vi "SA_SWEEP_TIME.vi"(0 "Session In":refnum<visa-resource-name>="TCPIP0::K-N90X0A-00005.local::hislip0::INSTR", 1 "RO(F)":bool, 2 "Skip(F)":bool, 11 "error in":errorcluster {"code" format="%.0x"}, 12 "SetTime(ms)":u16=1, 13 "Timeout":u32=3000) -> (4 "Session Out":refnum<visa-resource-name>, 10 "GetTime(ms)":dbl, 15 "error out":errorcluster {"code" format="%.0x"})   [LabVIEW 2018]
doc: "Launches the Instrument I/O Assistant, which you can use to communicate with message-based instruments and graphically parse the response. For example you can communicate with an instrument that uses a serial, Ethernet, or GPIB interface."
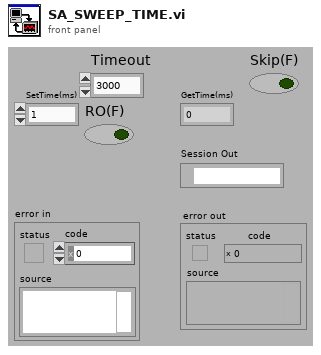
[diagram p1: front panel]
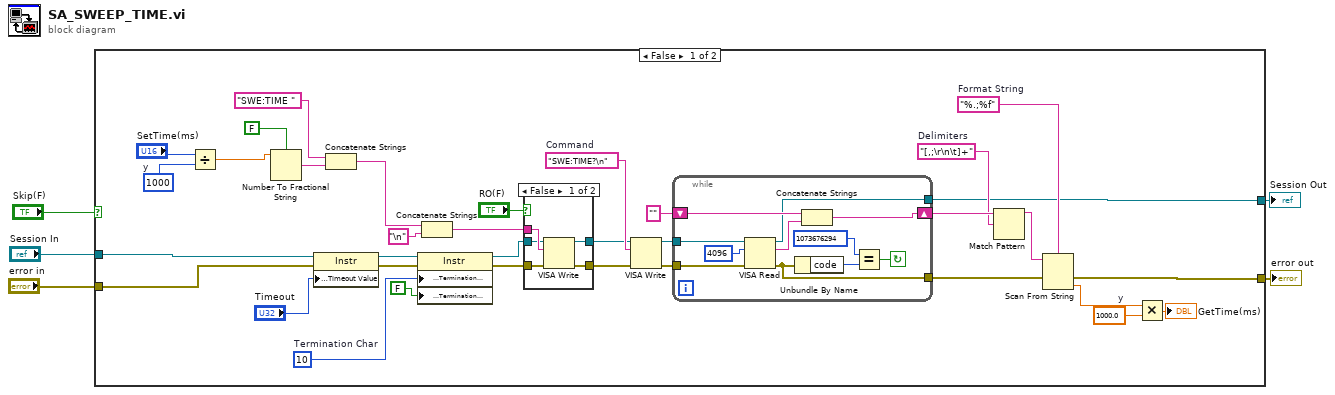
[diagram p0: block diagram]
diagram:
  n1 = case shown="False" "Skip(F)" {
    tunnel: "error in" -> [w40 w59]
    tunnel: "Session In" -> [w36 w60]
    tunnel: [w16 w59] -> w3
    tunnel: [w11 w60] -> w2
    frame False {
      w6 = 1000.0  # y
      w9 = u16 1000  # y
      w14 = "[,;\r\n\t]+"  # Delimiters
      w17 = "%.;%f"  # Format String
      w20 = "SWE:TIME?\n"  # Command
      w33 = u8 10  # Termination Char
      n2 = Divide(x="SetTime(ms)", y=w9) -> (x/y=w8:dbl)
      n3 = Number To Fractional String(use system decimal point (T)=FALSE, number=w8) -> (F-format string=w30:string)  [unwired: 2 in]
      n4 = property class="Instr"(reference=w36, error in=w40, "General Settings:Timeout Value"="Timeout") -> (reference out=w32:refnum<visa-resource-name>, error out=w35:errorcluster)
      n5 = Concatenate Strings("SWE:TIME " ("staticText"), w30) -> (w26:string)
      n6 = property class="Instr"(reference=w32, error in=w35, "Message Based Settings:Termination Character"=w33, "Message Based Settings:Termination Character Enable"=FALSE ("enable")) -> (reference out=w13:refnum<visa-resource-name>, error out=w34:errorcluster)
      n7 = Concatenate Strings(w26, "\n" ("StaticText")) -> (w27:string)
      n8 = case shown="False" "RO(F)" {
        tunnel: w34 -> [w45 w46]
        tunnel: [w44 w46] -> w28
        tunnel: w27 -> [w43 _]
        tunnel: w13 -> [w42 w47]
        tunnel: [w41 w47] -> w12
        frame False {
          n9 = VISA Write(VISA resource name=w42, write buffer=w43, error in (no error)=w45) -> (VISA resource name out=w41:refnum<visa-resource-name>, error out=w44:errorcluster)  [unwired: 1 out]
        }
        frame True {
        }
      }
      n10 = VISA Write(VISA resource name=w12, write buffer=w20, error in (no error)=w28) -> (VISA resource name out=w24:refnum<visa-resource-name>, error out=w23:errorcluster)  [unwired: 1 out]
      n11 = while {
        tunnel: w24 -> [w55]
        shift-right: [w49] -> w19
        shift-left: "" -> [w54]
        tunnel: w23 -> [w52]
        tunnel: [w51] -> w22
        tunnel: [w48] -> w11
        stop <- w50 continue-if-true
        n12 = VISA Read(VISA resource name=w55, byte count=u32 4096 ("byte count (0)"), error in (no error)=w52) -> (VISA resource name out=w48:refnum<visa-resource-name>, read buffer=w53:string, error out=w51:errorcluster)  [unwired: 1 out]
        n13 = Unbundle By Name(w51) -> ("code"=w57:i32)
        n14 = Concatenate Strings(w54, w53) -> (w49:string)
        n15 = Equal?(x=1073676294, y=w57) -> (x = y?=w50:bool)
      }
      n16 = Match Pattern(string=w19, regular expression=w14) -> (before substring=w18:string)  [unwired: 1 in, 3 out]
      n17 = Scan From String(format string=w17, input string=w18, error in=w22) -> (error out=w16:errorcluster, output 1=w15:dbl)  [unwired: 2 in, 2 out]
      n18 = Multiply(x=w15, y=w6) -> (x*y=→"GetTime(ms)":dbl)
    }
    frame True {
    }
  }
  "error out" <- w3
  "Session Out" <- w2
